vi "CH2_Comm.vi"() -> ()   [LabVIEW 2018]
uses:
  Stream/Stream.lvclass
  RxTx/RxTx.lvclass
  Stream/Stream.lvclass/Stream.ctl
panel:
  in  "RxTx.lvclass 2":refnum<class "RxTx.lvclass">
  in  "Stream.lvclass 2":refnum<class "Stream.lvclass">
  in  "RxTx.lvclass":refnum<class "RxTx.lvclass">
  in  "Stream.lvclass":refnum<class "Stream.lvclass">
  in  "Channel:":u16=2
  in  "IP:":string="localhost"
  # "Channel 1 Stream Communication"
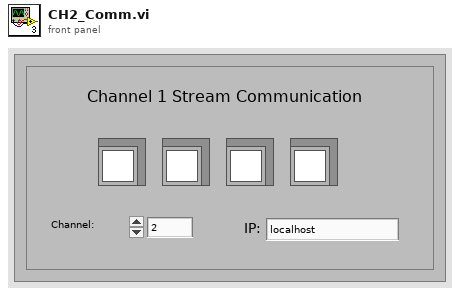
[diagram p1: front panel]
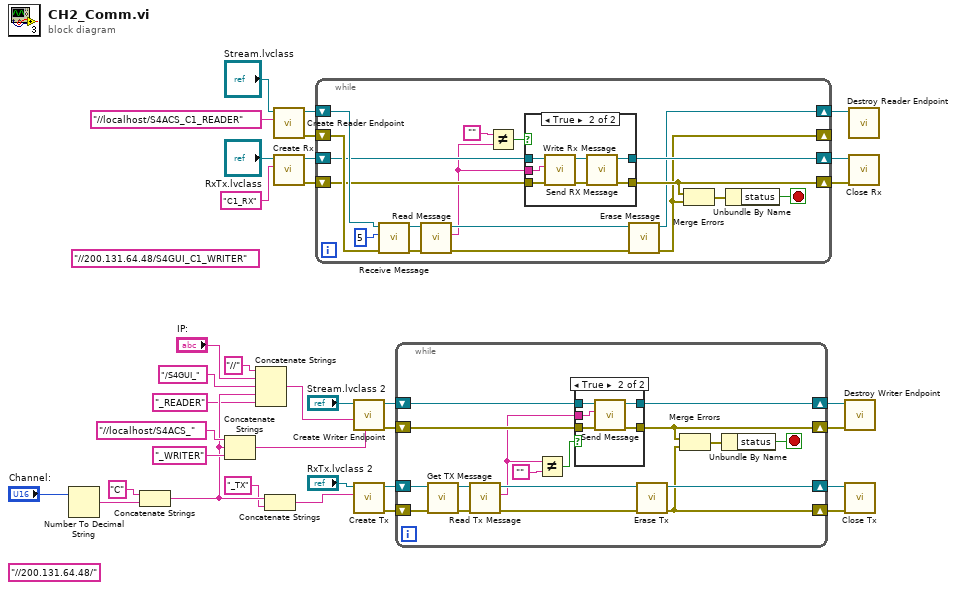
[diagram p0: block diagram]
diagram:
  (unwired) "//200.131.64.48/" ("Reader Name")
  (unwired) "//200.131.64.48/S4GUI_C1_WRITER" ("witer name")
  n1 = Number To Decimal String(number="Channel:") -> (decimal integer string=w10:string)  [unwired: 1 in]
  n2 = Concatenate Strings("C", w10) -> (w4:string)
  n3 = Concatenate Strings("//localhost/S4ACS_" ("reader name"), w4, "_WRITER" ("reader name")) -> (w5:string)
  n4 = Concatenate Strings("//" ("Reader Name"), "IP:", "/S4GUI_" ("Reader Name"), w4, "_READER" ("Reader Name")) -> (w2:string)
  n5 = Concatenate Strings(w4, "_TX" ("Reader Name")) -> (w8:string)
  n6 = call "Create Reader Endpoint.vi"("reader name"="//localhost/S4ACS_C1_READER", "Stream in"="Stream.lvclass") -> ("error out"=w32:errorcluster, "Stream out"=w33:refnum<class "Stream.lvclass">)  [unwired: 8 in]
  n7 = call "Create Rx.vi"("Reader Name"="C1_RX", "RxTx in"="RxTx.lvclass") -> ("error out"=w27:errorcluster, "RxTx out"=w28:refnum<class "RxTx.lvclass">)  [unwired: 8 in]
  n8 = while {
    shift-right: [w38] -> _
    shift-left: w32 -> [w52]
    shift-right: [w41] -> w31
    shift-left: w33 -> [w53]
    shift-right: [w45] -> w25
    shift-left: w27 -> [w49]
    shift-right: [w47] -> w26
    shift-left: w28 -> [w48]
    stop <- w36 stop-if-true
    n9 = call "Receive Message.vi"("error in (no error)"=w52, "timeout ms"=5, "Stream in"=w53) -> ("error out"=w50:errorcluster, "Stream out"=w51:refnum<class "Stream.lvclass">)  [unwired: 7 in]
    n10 = call "Read Message.vi"("error in (no error)"=w50, "Stream in"=w51) -> ("error out"=w40:errorcluster, "Message"=w37:string, "Stream out"=w39:refnum<class "Stream.lvclass">)  [unwired: 7 in]
    n11 = Not Equal?(x="", y=w37) -> (x != y?=w42:bool)
    n12 = case shown="True" w42 {
      tunnel: w49 -> [w54 w60]
      tunnel: w48 -> [w55 w59]
      tunnel: w37 -> [_ w58]
      tunnel: [w55 w57] -> w47
      tunnel: [w54 w56] -> w45
      frame False {
      }
      frame True {
        n13 = call "Write Rx Message.vi"("error in (no error)"=w60, "Rx Message"=w58, "RxTx in"=w59) -> ("error out"=w61:errorcluster, "RxTx out"=w62:refnum<class "RxTx.lvclass">)  [unwired: 7 in]
        n14 = call "Send RX Message.vi"("error in (no error)"=w61, "RxTx in"=w62) -> ("error out"=w56:errorcluster, "RxTx out"=w57:refnum<class "RxTx.lvclass">)  [unwired: 8 in]
      }
    }
    n15 = call "Erase Message.vi"("error in (no error)"=w40, "Stream in"=w39) -> ("error out"=w38:errorcluster, "Stream out"=w41:refnum<class "Stream.lvclass">)  [unwired: 8 in]
    n16 = Merge Errors(w45, w38) -> (w46:errorcluster)
    n17 = Unbundle By Name(w46) -> ("status"=w36:bool)
  }
  n18 = call "Create Writer Endpoint.vi"("writer name"=w5, "reader name"=w2, "Stream in"="Stream.lvclass 2") -> ("error out"=w17:errorcluster, "Stream out"=w19:refnum<class "Stream.lvclass">)  [unwired: 7 in]
  n19 = call "Create Tx.vi"("Writer Name"=w8, "RxTx in"="RxTx.lvclass 2") -> ("error out"=w22:errorcluster, "RxTx out"=w23:refnum<class "RxTx.lvclass">)  [unwired: 8 in]
  n20 = while {
    shift-right: [w72] -> w16
    shift-left: w17 -> [w74]
    shift-right: [w73] -> w24
    shift-left: w19 -> [w75]
    shift-right: [w67] -> w20
    shift-left: w22 -> [w76]
    shift-right: [w69] -> w21
    shift-left: w23 -> [w77]
    stop <- w63 stop-if-true
    n21 = call "Get TX Message.vi"("error in (no error)"=w76, "RxTx in"=w77) -> ("error out"=w78:errorcluster, "RxTx out"=w65:refnum<class "RxTx.lvclass">)  [unwired: 8 in]
    n22 = call "Read Tx Message.vi"("error in (no error)"=w78, "RxTx in"=w65) -> ("error out"=w68:errorcluster, "Tx Message"=w64:string, "RxTx out"=w70:refnum<class "RxTx.lvclass">)  [unwired: 7 in]
    n23 = Not Equal?(x=w64, y="") -> (x != y?=w66:bool)
    n24 = case shown="True" w66 {
      tunnel: w75 -> [w81 w86]
      tunnel: w74 -> [w80 w85]
      tunnel: [w81 w84] -> w73
      tunnel: w64 -> [_ w83]
      tunnel: [w80 w82] -> w72
      frame False {
      }
      frame True {
        n25 = call "Send Message.vi"("error in (no error)"=w85, "Message"=w83, "Stream in"=w86) -> ("error out"=w82:errorcluster, "Stream out"=w84:refnum<class "Stream.lvclass">)  [unwired: 7 in]
      }
    }
    n26 = call "Erase Tx.vi"("error in (no error)"=w68, "RxTx in"=w70) -> ("error out"=w67:errorcluster, "RxTx out"=w69:refnum<class "RxTx.lvclass">)  [unwired: 8 in]
    n27 = Merge Errors(w72, w67) -> (w79:errorcluster)
    n28 = Unbundle By Name(w79) -> ("status"=w63:bool)
  }
  n29 = call "Destroy Writer Endpoint.vi"("error in (no error)"=w16, "Stream in"=w24) -> ()  [unwired: 8 in, 2 out]
  n30 = call "Close Tx.vi"("error in (no error)"=w20, "RxTx in"=w21) -> ()  [unwired: 8 in, 2 out]
  n31 = call "Destroy Reader Endpoint.vi"("Stream in"=w31) -> ()  [unwired: 9 in, 2 out]
  n32 = call "Close Rx.vi"("error in (no error)"=w25, "RxTx in"=w26) -> ()  [unwired: 8 in, 2 out]
